vi "Write Input 2.vi"(8 "error in (no error)":errorcluster, 10 "Input 2":sgl, 11 "TECData in":refnum<class "TECData.lvclass">) -> (0 "error out":errorcluster, 3 "TECData out":refnum<class "TECData.lvclass">)   [LabVIEW 2014, in "TE Cooler.lvlib" / "TECData.lvclass"]
uses:
  TECData.lvclass
  TECData.lvclass/TECData.ctl
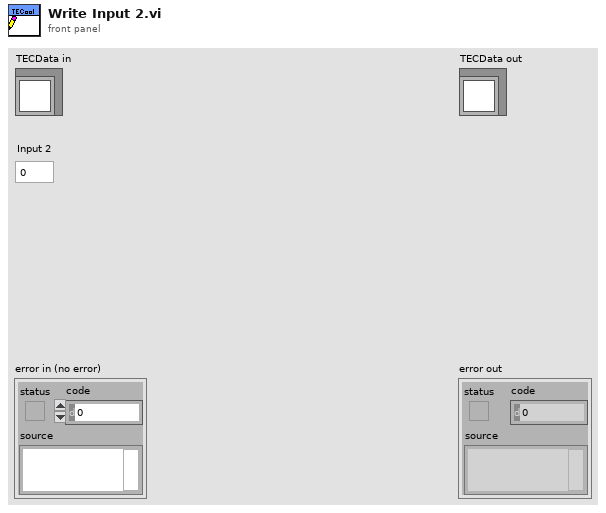
[diagram p1: front panel]
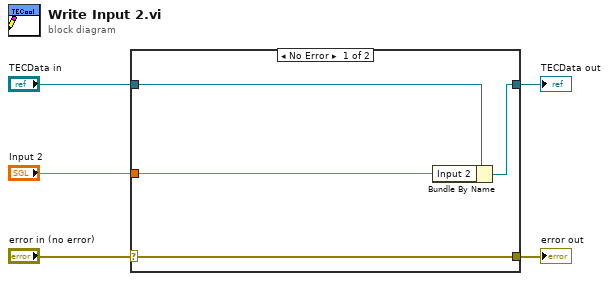
[diagram p0: block diagram]
diagram:
  n1 = case shown="No Error" "error in (no error)" {
    selector: "error in (no error)" -> [w9 w10]
    tunnel: [w9 w10] -> w4
    tunnel: [w7 w11] -> w2
    tunnel: "TECData in" -> [w8 w11]
    tunnel: "Input 2" -> [w6 _]
    frame No Error {
      n2 = Bundle By Name(cluster=w8, "Input 2"=w6) -> (w7:refnum<class "TECData.lvclass">)
    }
    frame Error {
    }
  }
  "error out" <- w4
  "TECData out" <- w2
